vi "SMO.UI.Embedded.Basic.TestLauncher.vi"() -> ()   [LabVIEW 2019, in "SMO.UI.Embedded.Basic.lvclass"]
uses:
  SMO.UI.Embedded.Basic.lvclass
  <vilib>/JKI/JKI SMO/SMO/Typedefs/SMOState --Enum.ctl
  C:/Program Files (x86)/National Instruments/LabVIEW 2019/vi.lib/JKI/JKI SMO/SMO/SMO.lvclass
  C:/Program Files (x86)/National Instruments/LabVIEW 2019/vi.lib/JKI/JKI SMO/SMO.UI/SMO.UI.lvclass
  <vilib>/JKI/JKI SMO/SMO/SMO.lvclass/SMO.ctl
  <vilib>/JKI/JKI SMO/SMO/Private/ReftoDVR--SMO.vi
  <vilib>/JKI/JKI SMO/SMO/SMO.lvclass
  <vilib>/JKI/JKI SMO/SMO.UI/SMO.UI.lvclass
panel:
  out "SMO State":T1
  out "error out":errorcluster
  in  "Stop":bool
  # "Embedded SMO Test Launcher"
  # "For Debugging (Please Ignore)"
  # "For instructions on how to use the JKI State Machine Objects, examples and video tutorials, visit:\nhttp://jki.net/state-machine-objects/\n\nJKI State Machine Objects™\nhttp://jki.net/state-machine-objects/\nCopyright (C) 2005-2015, JKI <info@jki.net>\nALL RIGHTS RESERVED"
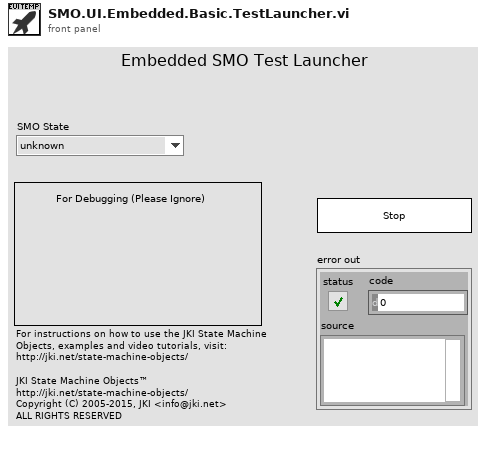
[diagram p1: front panel]
types:
  T1 = typedef "SMO.lvclass/SMOState --Enum.ctl" = enum16{"unknown", "Created", "Started", "Stopped"}
  T2 = typedef "SMO.lvclass/Public Events.ctl" = cluster{"Error":refnum<user-event>, "State":refnum<user-event>, "Reserve State":refnum<user-event>}
  T3 = cluster{"Event Registration Refnum":refnum<event-registration>}
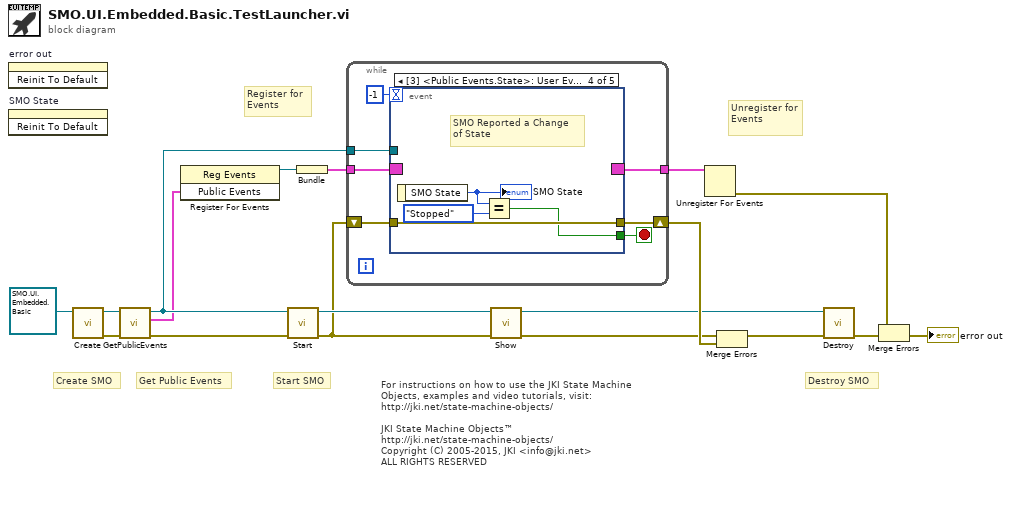
[diagram p0: block diagram]
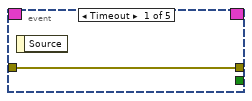
[diagram p2: hidden frame]
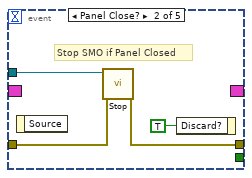
[diagram p3: hidden frame]
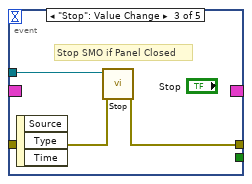
[diagram p4: hidden frame]
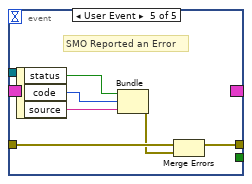
[diagram p5: hidden frame]
diagram:
  # "For instructions on how to use the JKI State Machine Objects, examples and video tutorials, visit:\nhttp://jki.net/state-machine-objects/\n\nJKI State Machine Objects™\nhttp://jki.net/state-machine-objects/\nCopyright (C) 2005-2015, JKI <info@jki.net>\nALL RIGHTS RESERVED"
  # "Get Public Events"
  # "Start SMO"
  # "Destroy SMO"
  # "Create SMO"
  # "Unregister for Events"
  # "Register for Events"
  n1 = invoke on="error out" class="Clust (strict)" method="Reinit To Default"() -> ()  [unwired: 3 in, 3 out]
  n2 = invoke on="SMO State" class="Enum (strict)" method="Reinit To Default"() -> ()  [unwired: 3 in, 3 out]
  n3 = call <vilib>:"Create.vi"("SMO"=refnum<class "SMO.UI.Embedded.Basic.lvclass"> refnum ("SMO.Template.lvclass")) -> ("error out"=w10:errorcluster, "SMO out"=w11:refnum<class "SMO.UI.Embedded.Basic.lvclass">)  [unwired: 8 in, 1 out]
  n4 = call <vilib>:"GetPublicEvents.vi"("error in (no error)"=w10, "SMO"=w11) -> ("error out"=w9:errorcluster, "Public Events"=w7:T2, "SMO out"=w8:refnum<class "SMO.UI.Embedded.Basic.lvclass">)  [unwired: 7 in]
  n5 = register-events(w7) -> (reference out=w6:refnum<event-registration>)  [unwired: 2 in, 1 out]
  n6 = call <vilib>:"Start.vi"("error in (no error)"=w9, "SMO"=w8) -> ("error out"=w3:errorcluster, "SMO out"=w5:refnum<class "SMO.UI.Embedded.Basic.lvclass">)  [unwired: 8 in]
  n7 = Bundle("Event Registration Refnum"=w6) -> (w17:T3)  [unwired: 1 in]
  n8 = while {
    shift-right: [w24] -> w16
    shift-left: w3 -> [w23]
    tunnel: w17 -> [w22]
    tunnel: [w21] -> w18
    tunnel: w8 -> [w20]
    stop <- w25 stop-if-true
    n9 = event shown="[3] <Public Events.State>: User Event" {
      selector: w22 -> [_ _ _ _ _]
      dyn-events: [_ _ _ _ _] -> w21
      timeout: -1 -> [_ _ _ _ _]
      tunnel: [_ _ _ w34 _] -> w25
      tunnel: w20 -> [_ w30 w33 _ _]
      tunnel: [w26 w29 w32 w37 w41] -> w24
      tunnel: w23 -> [w26 w28 w31 w37 w39]
      event Timeout {
        n10 = event-data() -> ()  [unwired: 1 in, 1 out]
      }
      event Panel Close? {
        # "Stop SMO if Panel Closed"
        n11 = event-data() -> ()  [unwired: 1 in, 1 out]
        n12 = call <vilib>:"Stop.vi"("error in (no error)"=w28, "SMO"=w30) -> ("error out"=w29:errorcluster)  [unwired: 8 in, 1 out]
        n13 = event-data("Discard?"=TRUE ("OK")) -> ()  [unwired: 1 in, 1 out]
      }
      event "Stop": Value Change {
        # "Stop SMO if Panel Closed"
        n14 = event-data() -> ()  [unwired: 1 in, 3 out]
        n15 = call <vilib>:"Stop.vi"("error in (no error)"=w31, "SMO"=w33) -> ("error out"=w32:errorcluster)  [unwired: 8 in, 1 out]
      }
      event User Event {
        # "SMO Reported a Change\nof State"
        n16 = event-data() -> ("SMO State"=w36:T1)  [unwired: 1 in]
        "SMO State" <- w36
        n17 = Equal?(x=w36, y=SMOState_--Enum."Stopped") -> (x = y?=w34:bool)
      }
      event User Event {
        # "SMO Reported an Error"
        n18 = event-data() -> ("status"=w40:bool, "code"=w43:i32, "source"=w42:string)  [unwired: 1 in]
        n19 = Bundle("status"=w40, "code"=w43, "source"=w42) -> (w38:errorcluster)  [unwired: 1 in]
        n20 = Merge Errors(w39, w38) -> (w41:errorcluster)
      }
    }
  }
  n21 = call <vilib>:"Show.vi"("error in (no error)"=w3, "SMO.UI"=w5) -> ("error out"=w2:errorcluster, "SMO.UI out"=w4:refnum<class "SMO.UI.Embedded.Basic.lvclass">)  [unwired: 8 in]
  n22 = Unregister For Events(event registration refnum=w18) -> (error out=w15:errorcluster)  [unwired: 1 in]
  n23 = Merge Errors(w2, w16) -> (w12:errorcluster)
  n24 = call <vilib>:"Destroy.vi"("error in (no error)"=w12, "SMO"=w4) -> ("error out"=w13:errorcluster)  [unwired: 9 in]
  n25 = Merge Errors(w15, w13) -> (→"error out":errorcluster)
